vi "Execute-RT-Cert.vi"   [LabVIEW 2014]
uses:
  <vilib>/Utility/error.llb/DialogType.ctl
  <vilib>/Wiresmith Technology/LabVIEW CLI/CLI Class/CLI.lvclass
types:
  T1 = typedef "DialogType.ctl" = u16
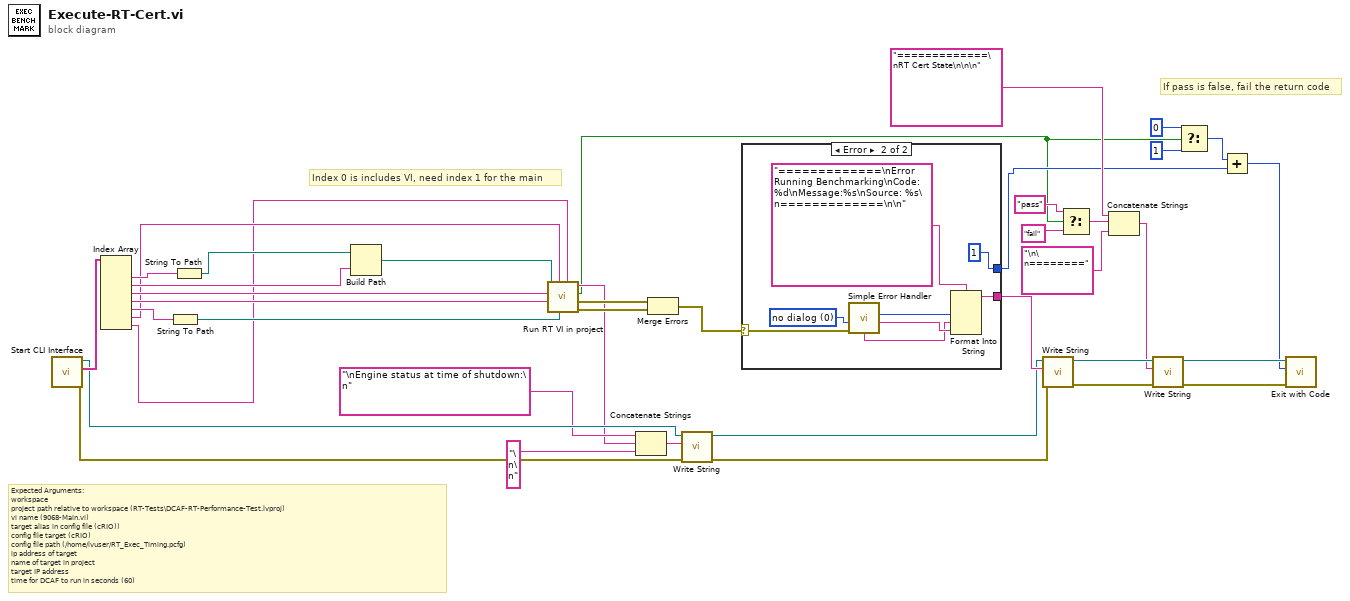
[diagram p0: block diagram]
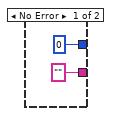
[diagram p2: hidden frame]
diagram:
  # "If pass is false, fail the return code"
  # "Index 0 is includes VI, need index 1 for the main"
  # "Expected Arguments:\nworkspace \nproject path relative to workspace (RT-Tests\\DCAF-RT-Performance-Test.lvproj)\nvi name (9068-Main.vi)\ntarget alias in config file (cRIO))\nconfig file target (cRIO)\nconfig file path (/home/lvuser/RT_Exec_Timing.pcfg)\nip address of target\nname of target in project\ntarget IP address\ntime for DCAF to run in seconds (60)"
  n1 = call <vilib>:"Start CLI Interface.vi"() -> ("error out"=w22:errorcluster, "Custom Parameters"=w39:string[], "CLI out"=w25:refnum<class "CLI.lvclass">)  [unwired: 9 in]
  n2 = Index Array(array=w39) -> (element #1=w27:string, element #2=w35:string, element #3=w33:string, element #4=w32:string, element #5=w37:string, element #6=w18:string, element #7=w17:string)  [unwired: 7 in]
  n3 = String To Path(string=w37) -> (path=w31:path)
  n4 = String To Path(string=w27) -> (path=w36:path)
  n5 = Build Path(base path=w36, name or relative path=w35) -> (appended path=w34:path)
  n6 = call "Run RT VI in project.vi"("project target"=w17, "configuration file path"=w31, "ip address"=w18, "target alias"=w32, "vi name"=w33, "Project Path"=w34) -> ("error out"=w30:errorcluster, "invoked VI error out"=w29:errorcluster, "pass"=w2:bool, "engine status"=w19:string)  [unwired: 2 in]
  n7 = Concatenate Strings("\nEngine status at time of shutdown:\n" ("string"), w19, "\n\n" ("string")) -> (w26:string)
  n8 = Merge Errors(w29, w30) -> (w28:errorcluster)
  n9 = call <vilib>:"Write String.vi"("error in (no error)"=w22, "Text to Write"=w26, "CLI in"=w25) -> ("error out"=w23:errorcluster, "CLI out"=w24:refnum<class "CLI.lvclass">)  [unwired: 7 in]
  n10 = case shown="Error" w28 {
    selector: w28 -> [_ w46]
    tunnel: ["" w42] -> w38
    tunnel: [0 ("Exit Code (0)") 1 ("Exit Code (0)")] -> w6
    frame No Error {
    }
    frame Error {
      w47 = T1 0 items=["no dialog", "OK message", "continue or stop message", "OK message + warnings", "continue/stop + warnings"] ("type of dialog (OK msg:1)")
      n11 = call <vilib>:"Simple Error Handler.vi"("type of dialog (OK msg:1)"=w47, "error in (no error)"=w46) -> ("code out"=w45:i32, "source out"=w44:string, "message"=w43:string)  [unwired: 3 in, 2 out]
      n12 = Format Into String(format string="=============\nError Running Benchmarking\nCode: %d\nMessage:%s\nSource: %s\n=============\n\n", w45, w43, w44) -> (resulting string=w42:string)  [unwired: 2 in, 1 out]
    }
  }
  n13 = call <vilib>:"Write String.vi"("error in (no error)"=w23, "Text to Write"=w38, "CLI in"=w24) -> ("error out"=w10:errorcluster, "CLI out"=w11:refnum<class "CLI.lvclass">)  [unwired: 7 in]
  n14 = Select(t="pass" ("format string"), s=w2, f="fail" ("format string")) -> (s? t:f=w16:string)
  n15 = Concatenate Strings("=============\nRT Cert State\n\n\n" ("format string"), w16, "\n\n========" ("string")) -> (w7:string)
  n16 = call <vilib>:"Write String.vi"("error in (no error)"=w10, "Text to Write"=w7, "CLI in"=w11) -> ("error out"=w8:errorcluster, "CLI out"=w9:refnum<class "CLI.lvclass">)  [unwired: 7 in]
  n17 = Select(t=0 ("Exit Code (0)"), s=w2, f=1 ("Exit Code (0)")) -> (s? t:f=w5:i32)
  n18 = Add(x=w5, y=w6) -> (x+y=w1:i32)
  n19 = call <vilib>:"Exit with Code.vi"("error in (no error)"=w8, "Exit Code (0)"=w1, "CLI in"=w9) -> ()  [unwired: 8 in, 1 out]
